vi "Servo MSMT LTE Configure Measure Step.vi"(8 "error in (no error)":errorcluster, 9 "Standard":string, 11 "Servo MSMT in":refnum<class "Servo MSMT.lvclass">) -> (0 "error out":errorcluster, 3 "Servo MSMT out":refnum<class "Servo MSMT.lvclass">)   [LabVIEW 2018, in "Servo MSMT.lvlib" / "Servo MSMT.lvclass"]
uses:
  Servo MSMT.lvclass
  C:/Sequence Automation/Plugins/Measurement Interface.lvlibp/Measurement Interface.lvclass
  Plugins/Measurement Interface.lvlibp/Private Methods/Measurement Name/Read Measurement Name.vi
  Plugins/TestStand API Tools (TSAT).lvlibp/Step Actions/TSAT Step Actions.lvlib
  Plugins/Measurement Interface.lvlibp/Measurement Interface.lvclass
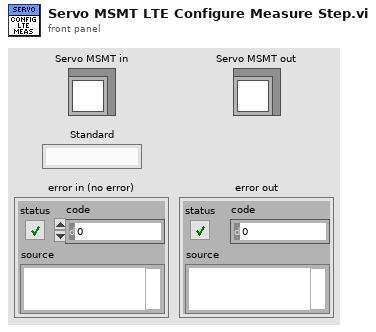
[diagram p1: front panel]
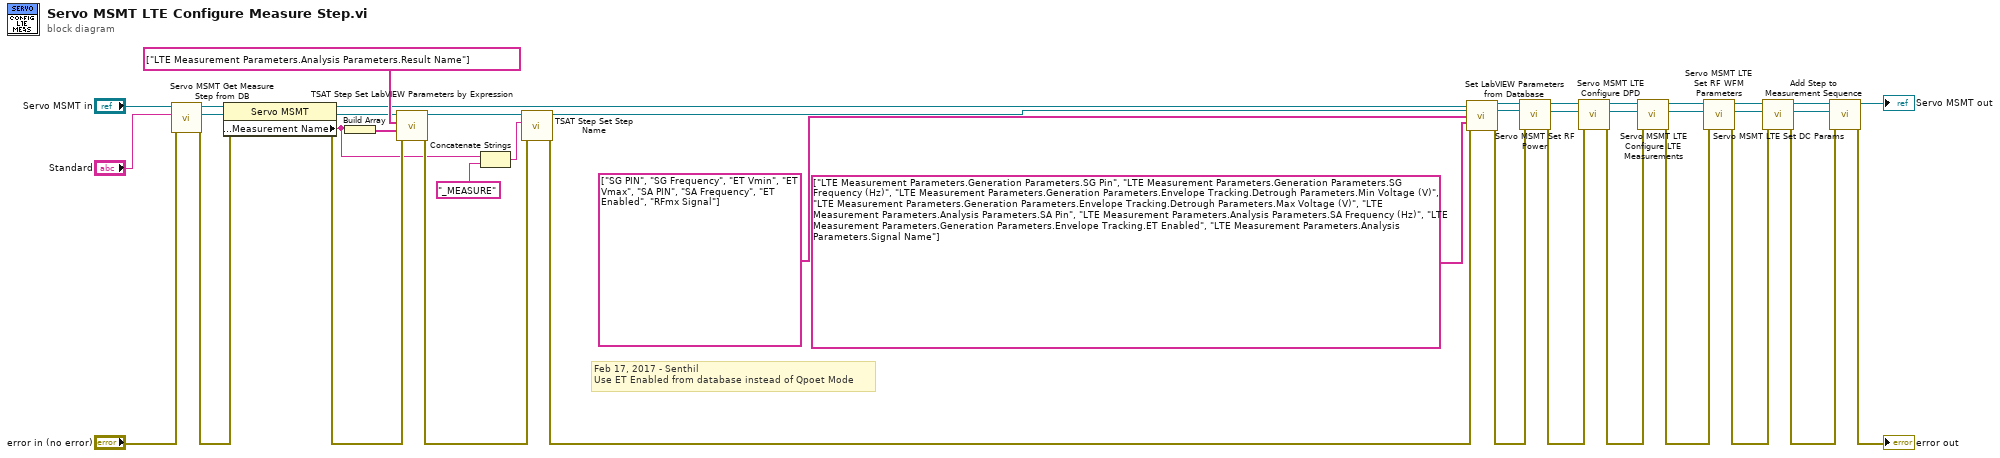
[diagram p0: block diagram]
diagram:
  # "Feb 17, 2017 - Senthil\nUse ET Enabled from database instead of Qpoet Mode"
  n1 = call "Servo MSMT Get Measure Step from DB.vi"("error in (no error)"="error in (no error)", "Standard"="Standard", "Servo MSMT in"="Servo MSMT in") -> ("error out"=w36:errorcluster, "Step Out"=w35:refnum<k7>, "Servo MSMT out"=w20:refnum<class "Servo MSMT.lvclass">)  [unwired: 6 in]
  n2 = property class="Servo MSMT"(reference=w20, error in=w36) -> (reference out=w19:refnum<class "Servo MSMT.lvclass">, error out=w21:errorcluster, "Public Methods:Measurement Name"=w1:string)
  n3 = Build Array(w1) -> (w38:string[])
  n4 = call "TSAT Step Set LabVIEW Parameters by Expression.vi"("Error In"=w21, "Value Expressions"=w38, "Parameters to Set"=string[] ["LTE Measurement Parameters.Analysis Parameters.Result Name"], "Step In"=w35) -> ("Error Out"=w3:errorcluster, "Step Out"=w6:refnum<k7>)  [unwired: 6 in]
  n5 = Concatenate Strings(w1, "_MEASURE" ("string")) -> (w4:string)
  n6 = call "TSAT Step Set Step Name.vi"("Error In"=w3, "Name"=w4, "Step In"=w6) -> ("Error Out"=w2:errorcluster, "Step Out"=w5:refnum<k7>)  [unwired: 7 in]
  n7 = call "Set LabVIEW Parameters from Database.vi"("Measurement Interface in"=w19, "Step In"=w5, "Dictionary Keys"=string[] ["SG PIN", "SG Frequency", "ET Vmin", "ET Vmax", "SA PIN", "SA Frequency", "ET Enabled", "RFmx Signal"] ("Database Keys"), "LabVIEW Parameter Mapping"=string[] ["LTE Measurement Parameters.Generation Parameters.SG Pin", "LTE Measurement Parameters.Generation Parameters.SG Frequency (Hz)", "LTE Measurement Parameters.Generation Parameters.Envelope Tracking.Detrough Parameters.Min Voltage (V)", "LTE Measurement Parameters.Generation Parameters.Envelope Tracking.Detrough Parameters.Max Voltage (V)", "LTE Measurement Parameters.Analysis Parameters.SA Pin", "LTE Measurement Parameters.Analysis Parameters.SA Frequency (Hz)", "LTE Measurement Parameters.Generation Parameters.Envelope Tracking.ET Enabled", "LTE Measurement Parameters.Analysis Parameters.Signal Name"] ("Database Keys"), "error in (no error)"=w2) -> ("Measurement Interface out"=w17:refnum<class "Servo MSMT.lvclass">, "Step Out"=w16:refnum<k7>, "error out"=w26:errorcluster)  [unwired: 8 in]
  n8 = call-dynamic "Servo MSMT Set RF Power.vi"("error in (no error)"=w26, "Step In"=w16, "Servo MSMT in"=w17) -> ("error out"=w18:errorcluster, "Step Out"=w9:refnum<k7>, "Servo MSMT out"=w11:refnum<class "Servo MSMT.lvclass">)  [unwired: 6 in]
  n9 = call "Servo MSMT LTE Configure DPD.vi"("error in (no error)"=w18, "Step In"=w9, "Servo MSMT in"=w11) -> ("error out"=w12:errorcluster, "Step Out"=w8:refnum<k7>, "Servo MSMT out"=w10:refnum<class "Servo MSMT.lvclass">)  [unwired: 6 in]
  n10 = call "Servo MSMT LTE Configure LTE Measurements.vi"("error in (no error)"=w12, "Step In"=w8, "Servo MSMT in"=w10) -> ("error out"=w15:errorcluster, "Step Out"=w13:refnum<k7>, "Servo MSMT out"=w14:refnum<class "Servo MSMT.lvclass">)  [unwired: 6 in]
  n11 = call "Servo MSMT LTE Set RF WFM Parameters.vi"("error in (no error)"=w15, "Step In"=w13, "Servo MSMT in"=w14) -> ("error out"=w27:errorcluster, "Step Out"=w30:refnum<k7>, "Servo MSMT out"=w29:refnum<class "Servo MSMT.lvclass">)  [unwired: 6 in]
  n12 = call "Servo MSMT LTE Set DC Params.vi"("error in (no error)"=w27, "Step In"=w30, "Servo MSMT in"=w29) -> ("error out"=w28:errorcluster, "Step Out"=w34:refnum<k7>, "Servo MSMT out"=w32:refnum<class "Servo MSMT.lvclass">)  [unwired: 6 in]
  n13 = call "Add Step to Measurement Sequence.vi"("error in (no error)"=w28, "Step to Add"=w34, "Measurement Interface in"=w32) -> ("error out"=→"error out":errorcluster, "Measurement Interface out"=→"Servo MSMT out":refnum<class "Servo MSMT.lvclass">)  [unwired: 7 in]
